vi "Get Input Volume.vi"(7 "Mode (F = Mul / T = dB)":bool, 8 "error in (no error)":errorcluster, 10 "Input Name":string, 11 "OBS in":refnum<class "OBS.lvclass">) -> (0 "error out":errorcluster, 2 "Volume":dbl, 3 "OBS out":refnum<class "OBS.lvclass">)   [LabVIEW 2020, in "obs-websocket.lvlib" / "OBS.lvclass"]
uses:
  OBS.lvclass
  OBS.lvclass/OBS.ctl
  GetInputVolume/GetInputVolume.lvclass
  RGetInputVolume/RGetInputVolume.lvclass
  C:/dev/lv20CE/lv-obs-websocket/obs-websocket-lv/Response/Response.lvclass
  C:/dev/lv20CE/lv-obs-websocket/obs-websocket-lv/Server Message/Server Message.lvclass
  C:/dev/lv20CE/lv-obs-websocket/obs-websocket-lv/Message/Message.lvclass
  C:/dev/lv20CE/lv-obs-websocket/obs-websocket-lv/RGetInputVolume/RGetInputVolume.lvclass
  C:/dev/lv20CE/lv-obs-websocket/obs-websocket-lv/Request/Request.lvclass
  C:/dev/lv20CE/lv-obs-websocket/obs-websocket-lv/Client Message/Client Message.lvclass
  C:/dev/lv20CE/lv-obs-websocket/obs-websocket-lv/GetInputVolume/GetInputVolume.lvclass
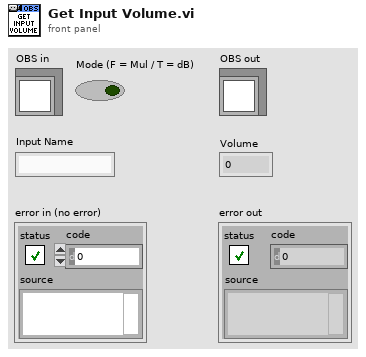
[diagram p1: front panel]
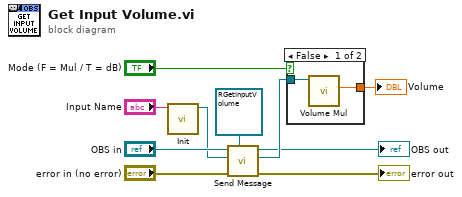
[diagram p0: block diagram]
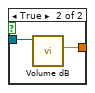
[diagram p2: hidden frame]
diagram:
  n1 = call "Init.vi"("Input Name"="Input Name") -> ("GetInputVolume out"=w7:refnum<class "GetInputVolume.lvclass">)  [unwired: 9 in, 1 out]
  n2 = call "Send Message.vi"("Response Type (None)"=refnum<class "RGetInputVolume.lvclass"> refnum ("obs-websocket-lv.lvlib:RGetInputVolume.lvclass"), "error in (no error)"="error in (no error)", "Client Message"=w7, "OBS in"="OBS in") -> ("error out"=→"error out":errorcluster, "Response Type (None)"=w5:refnum<class "RGetInputVolume.lvclass">, "OBS in"=→"OBS out":refnum<class "OBS.lvclass">)  [unwired: 4 in, 1 out]
  n3 = case shown="False" "Mode (F = Mul / T = dB)" {
    tunnel: w5 -> [w12 w14]
    tunnel: [w11 w13] -> w3
    frame False {
      n4 = call "Volume Mul.vi"("RGetInputVolume in"=w12) -> ("Volume Mul"=w11:dbl)  [unwired: 8 in, 2 out]
    }
    frame True {
      n5 = call "Volume dB.vi"("RGetInputVolume in"=w14) -> ("Volume dB"=w13:dbl)  [unwired: 8 in, 2 out]
    }
  }
  "Volume" <- w3
